vi "Interface_Dispatch_Process Module.vi"(8 "error in (no error)":errorcluster, 10 "TagBus DVR":refnum<data-value>, 11 "Interface_Dispatch in":refnum<class "Interface_Dispatch.lvclass">) -> (0 "error out":errorcluster, 2 "TagBus DVR out":refnum<data-value>, 3 "Interface_Dispatch out":refnum<class "Interface_Dispatch.lvclass">)   [LabVIEW 2015, in "Interface_Dispatch.lvclass"]
uses:
  Interface_Dispatch.lvclass
  TagBus/TagBus.lvclass
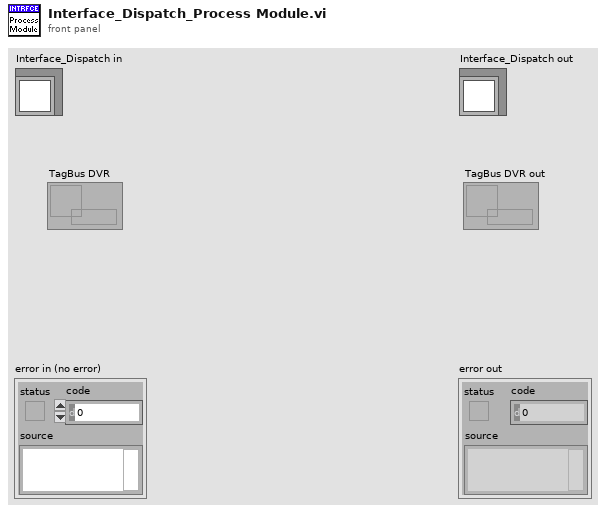
[diagram p1: front panel]
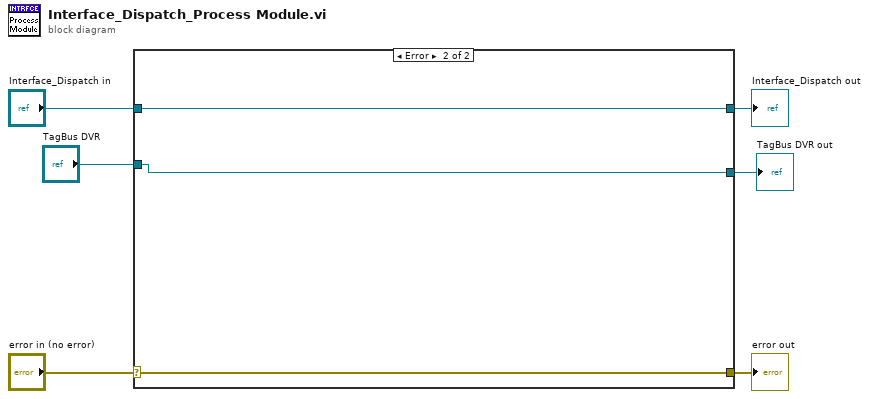
[diagram p0: block diagram]
diagram:
  n1 = case shown="Error" "error in (no error)" {
    selector: "error in (no error)" -> [w8 w12]
    tunnel: [w8 w12] -> w5
    tunnel: [w9 w11] -> w3
    tunnel: "Interface_Dispatch in" -> [w9 w11]
    tunnel: [w7 w10] -> w2
    tunnel: "TagBus DVR" -> [w7 w10]
    frame No Error {
      # "Wire the error cluster across even in the \"No Error\"\ncase so that warnings get propagated."
    }
    frame Error {
    }
  }
  "error out" <- w5
  "Interface_Dispatch out" <- w3
  "TagBus DVR out" <- w2
